vi "Initialize Session.vi"(8 "error in":errorcluster, 10 "shared resources":refnum<class "Shared Resources.lvclass">, 11 "Rx Execution Unit Implementation in":refnum<class "Rx Execution Unit.lvclass">) -> (0 "error out":errorcluster, 3 "Rx Execution Unit Implementation out":refnum<class "Rx Execution Unit.lvclass">)   [LabVIEW 2020, in "afdx_custom_device Engine.lvlib" / "Implementation.lvlib" / "Rx Execution Unit.lvclass"]
uses:
  Rx Execution Unit.lvclass
  AIM LabVIEW src/src/AIM664LV.lvlib
  AIM LabVIEW src/src/_polimorphicInstances/session/Fdx Create Session (RX-Monitor).vi
  Interfaces/Shared Resources/Shared Resources.lvclass
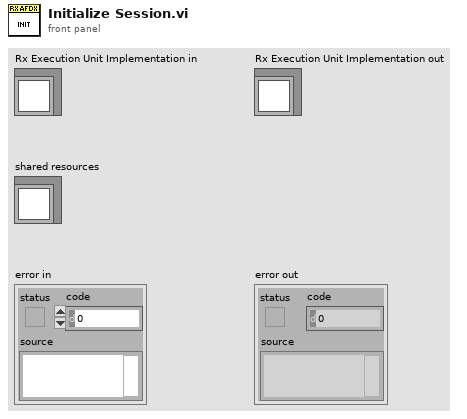
[diagram p1: front panel]
types:
  T1 = typedef "channel_settings_rx.ctl" = cluster{"Cluster":T2, "Rx Board":dbl, "Rx Port":dbl}
  T2 = typedef "AIM664LV.lvlib/session_monitor_config.ctl" = cluster{"DefaultCronoMode":u32, "GlbMonBufferSizeIn":u32}
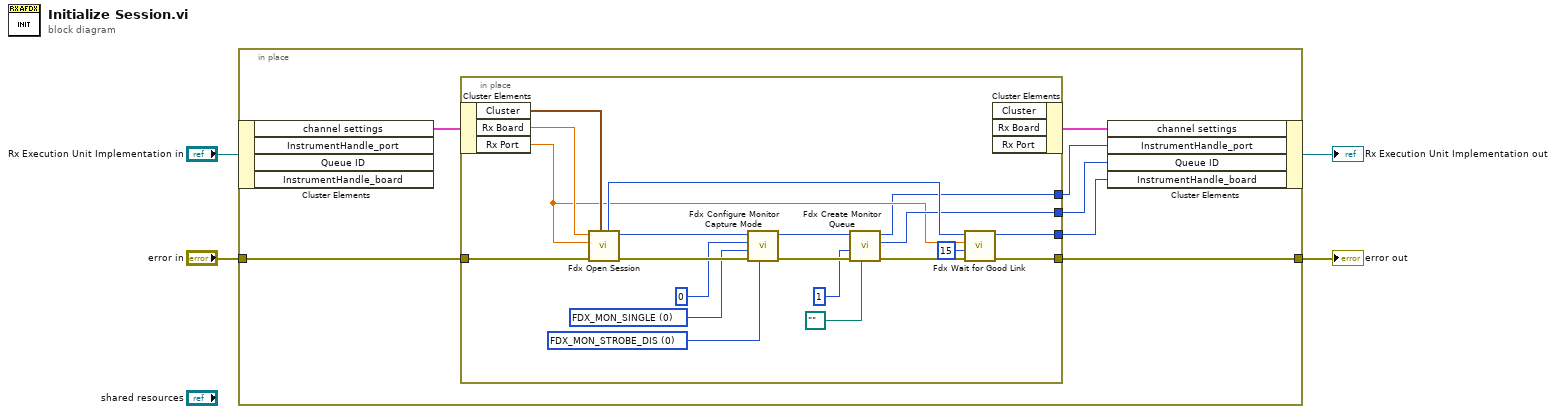
[diagram p0: block diagram]
diagram:
  n1 = in-place {
    in-place-border: "error in" -> [w10]
    in-place-border: [w8] -> w1
    n2 = in-place-cluster #1("Rx Execution Unit Implementation in") -> ("channel settings"=w11:T1)  [unwired: 3 out]
    n3 = in-place {
      in-place-border: w10 -> [w30]
      in-place-border: [w18] -> w8
      in-place-border: [w17] -> w7
      in-place-border: [w15] -> w6
      in-place-border: [w12] -> w5
      w22 = u32 0 items=["FDX_MON_STROBE_DIS", "FDX_MON_STROBE_STOP", "FDX_MON_STROBE_START"] ("Strobe")
      w23 = u32 0 items=["FDX_MON_SINGLE ", "FDX_MON_CONTINUOUS", "FDX_MON_SELECTIVE", "FDX_MON_RECORDING", "FDX_MON_REROS", "FDX_MON_HMU"] ("CaptureMode")
      n4 = in-place-cluster #2(w11) -> ("Cluster"=w28:T2, "Rx Board"=w31:dbl, "Rx Port"=w14:dbl)
      n5 = call-poly "Fdx Open Session.vi"("MonitorConfig"=w28, "error in (no error)"=w30, "port"=w14, "board"=w31) -> ("error out"=w29:errorcluster, "InstrumentHandle_port out"=w25:u32, "InstrumentHandle_board out"=w16:u32)  [unwired: 2 in, 3 out]
      n6 = call "Fdx Configure Monitor Capture Mode.vi"("Strobe"=w22, "error in (no error)"=w29, "CaptureMode"=w23, "TriggerPosition"=u32 0, "InstrumentHandle_port in"=w25) -> ("error out"=w27:errorcluster, "InstrumentHandle_port out"=w21:u32)  [unwired: 5 in]
      n7 = call "Fdx Create Monitor Queue.vi"("RecordingFileName"=path "", "error in (no error)"=w27, "MaxFileSize MB (1)"=u32 1, "InstrumentHandle_port in"=w21) -> ("error out"=w26:errorcluster, "QueueIdOut"=w15:u32, "InstrumentHandle_port out"=w12:u32)  [unwired: 4 in, 1 out]
      n8 = call "Fdx Wait for Good Link.vi"("error in"=w26, "timeout s(10)"=u32 15, "port id"=w14, "InstrumentHandle_board in"=w16) -> ("error out"=w18:errorcluster, "InstrumentHandle_board out"=w17:u32)  [unwired: 4 in, 2 out]
      n9 = in-place-cluster #2() -> (w9:T1)  [unwired: 3 in]
    }
    n10 = in-place-cluster #1("channel settings"=w9, "InstrumentHandle_port"=w5, "Queue ID"=w6, "InstrumentHandle_board"=w7) -> (→"Rx Execution Unit Implementation out":refnum<class "Rx Execution Unit.lvclass">)
  }
  "error out" <- w1
